vi "Shutdown.vi"(8 "error in (no error)":errorcluster, 11 "Instruments in":refnum<class "Instruments.lvclass">) -> (0 "error out":errorcluster, 3 "Instruments out":refnum<class "Instruments.lvclass">)   [LabVIEW 2023, in "Instruments.lvlib" / "Instruments.lvclass"]
doc: "<b>Shutdown</b>\nThis routine is implemented in the stop actor override -> as a result, it is not necessary to call shutdown anywhere else, and any methods that need to be called prior to stop actor core can be implemented here.\n\n<b>Engine</b> - No methods implemented at the engine level\n\n<b>Managed Actor</b> This routine transmits a stop core to all subordinate actors"
uses:
  Library/Instruments.lvclass
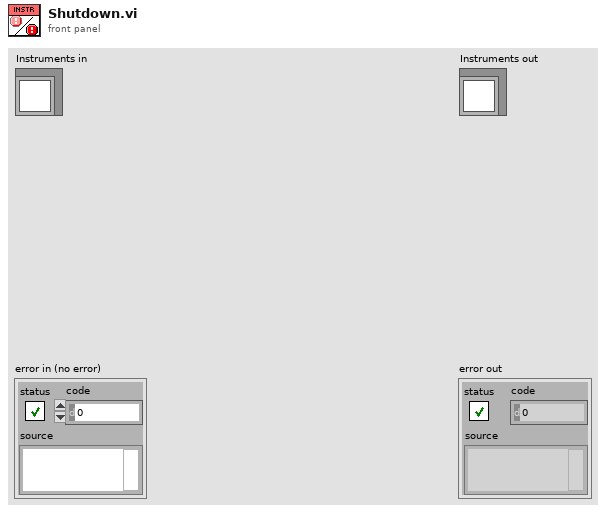
[diagram p1: front panel]
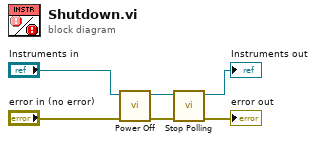
[diagram p0: block diagram]
diagram:
  n1 = call-dynamic "Power Off.vi"("error in (no error)"="error in (no error)", "Instruments in"="Instruments in") -> ("error out"=w1:errorcluster, "Instruments out"=w2:refnum<class "Instruments.lvclass">)  [unwired: 8 in]
  n2 = call "Stop Polling.vi"("error in (no error)"=w1, "Instruments in"=w2) -> ("error out"=→"error out":errorcluster, "Instruments out"=→"Instruments out":refnum<class "Instruments.lvclass">)  [unwired: 8 in]
